vi "AMI1700_meas_he_lev.vi"(7 "mode":enum16{"CONT", "HOLD"}(ring) caption="Readout Mode", 8 "error in":errorcluster, 11 "VISA in":refnum<visa-resource-name>) -> (0 "error out":errorcluster, 1 "level":dbl, 2 "status":bool, 3 "VISA out":refnum<visa-resource-name>, 4 "ADC2":string, 6 "LEV":string)   [LabVIEW 2019]
uses:
  <vilib>/Instr/_visa.llb/VISA Flush IO Buffer Mask.ctl
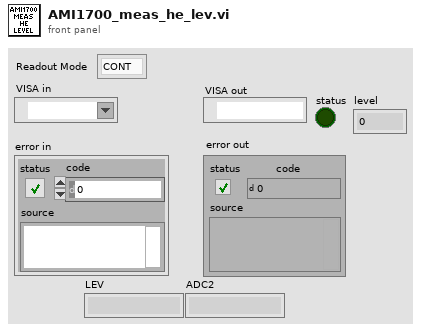
[diagram p1: front panel]
types:
  T1 = typedef "VISA Flush IO Buffer Mask.ctl" = u16
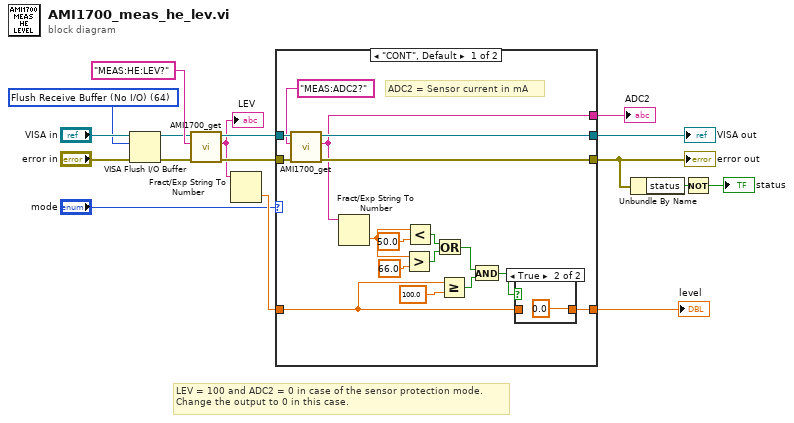
[diagram p0: block diagram]
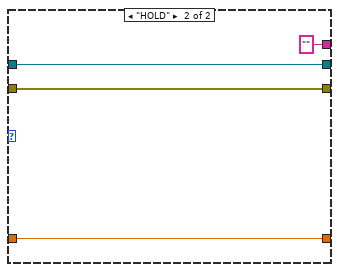
[diagram p3: hidden frame]
diagram:
  w1 = T1 64 items=["Flush Receive Buffer"=16, "Write Transmit Buffer to Device"=32, "Flush Receive Buffer (No I/O)"=64, "Flush Transmit Buffer"=128] ("Mask")
  # "LEV = 100 and ADC2 = 0 in case of the sensor protection mode.\nChange the output to 0 in this case."
  n1 = VISA Flush I/O Buffer(VISA resource name="VISA in", mask (16)=w1, error in (no error)="error in") -> (VISA resource name out=w4:refnum<visa-resource-name>, error out=w2:errorcluster)
  n2 = call "AMI1700_get.vi"("error in"=w2, "string in"="MEAS:HE:LEV?" ("string"), "VISA in"=w4) -> ("error out"=w14:errorcluster, "string out"=w13:string, "VISA out"=w16:refnum<visa-resource-name>)  [unwired: 6 in]
  "LEV" <- w13
  n3 = Fract/Exp String To Number(string=w13) -> (number=w12:dbl)  [unwired: 3 in, 1 out]
  n4 = case shown="\"CONT\", Default" "mode" {
    tunnel: w16 -> [w34 w40]
    tunnel: [w33 w40] -> w15
    tunnel: w14 -> [w32 w39]
    tunnel: w12 -> [w22 w38]
    tunnel: [w21 w38] -> w11
    tunnel: [w20 w39] -> w10
    tunnel: [w18 "" ("string out")] -> w6
    frame "CONT", Default {
      # "ADC2 = Sensor current in mA"
      n5 = call "AMI1700_get.vi"("error in"=w32, "string in"="MEAS:ADC2?" ("string"), "VISA in"=w34) -> ("error out"=w20:errorcluster, "string out"=w18:string, "VISA out"=w33:refnum<visa-resource-name>)  [unwired: 6 in]
      n6 = Fract/Exp String To Number(string=w18) -> (number=w27:dbl)  [unwired: 3 in, 1 out]
      n7 = Greater?(x=w27, y=66.0) -> (0:w28:bool)
      n8 = Less?(x=w27, y=50.0) -> (x < y?=w29:bool)
      n9 = Or(x=w29, y=w28) -> (x .or. y?=w25:bool)
      n10 = Greater Or Equal?(x=w22, y=100.0) -> (x >= y?=w24:bool)
      n11 = And(x=w25, y=w24) -> (x .and. y?=w23:bool)
      n12 = case shown="True" w23 {
        tunnel: [w35 0.0] -> w21
        tunnel: w22 -> [w35 _]
        frame False {
        }
        frame True {
        }
      }
    }
    frame "HOLD" {
    }
  }
  "VISA out" <- w15
  "error out" <- w10
  "level" <- w11
  "ADC2" <- w6
  n13 = Unbundle By Name(w10) -> ("status"=w9:bool)
  n14 = Not(x=w9) -> (.not. x?=→"status":bool)
